vi "onenote_dialog_Fit_image_max_size.vi"(8 "error in (no error)":errorcluster, 10 "image size (pixels)":cluster{"x":i16, "y":i16}, 11 "Picture Refnum":refnum<vi>) -> (0 "error out":errorcluster)   [LabVIEW 2016]
uses:
  <vilib>/Utility/miscctls.llb/LVBoundsTypeDef.ctl
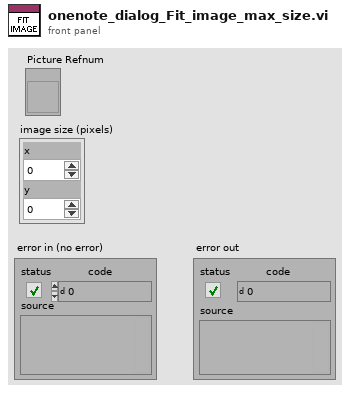
[diagram p1: front panel]
types:
  T1 = typedef "LVBoundsTypeDef.ctl" = cluster{"Width":u32, "Height":u32}
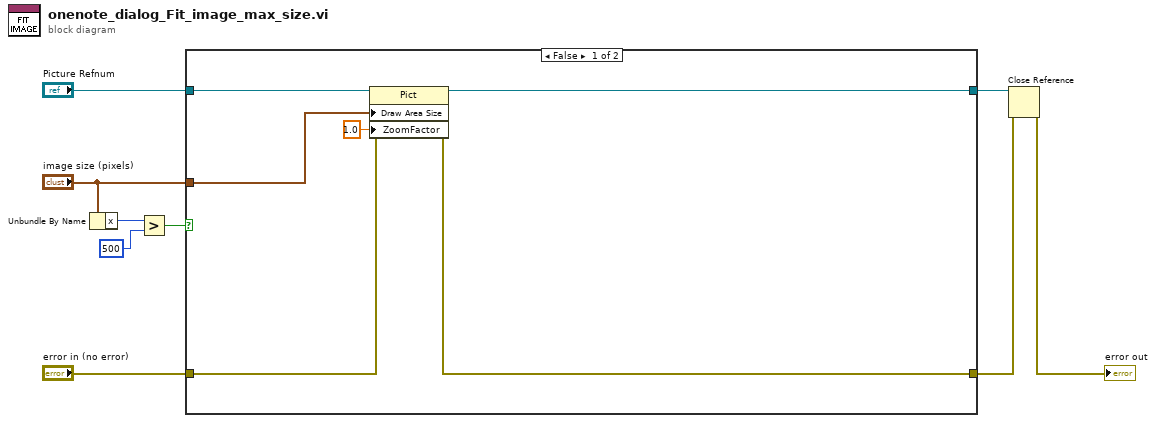
[diagram p0: block diagram]
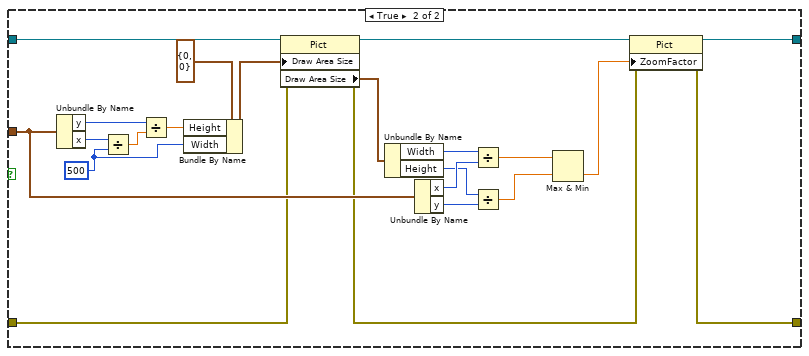
[diagram p2: hidden frame]
diagram:
  n1 = Unbundle By Name("image size (pixels)") -> ("x"=w9:i16)
  n2 = Greater?(x=w9, y=i16 500) -> (0:w7:bool)
  n3 = case shown="False" w7 {
    tunnel: "error in (no error)" -> [w12 w23]
    tunnel: "Picture Refnum" -> [w15 w37]
    tunnel: [w11 w17] -> w1
    tunnel: "image size (pixels)" -> [w14 w29]
    tunnel: [w10 w16] -> w3
    frame False {
      n4 = property class="Pict"(reference=w15, error in=w12, "Draw Area Size"=w14, "ZoomFactor"=sgl 1.0 ("Zoom Factor")) -> (reference out=w10:refnum<vi>, error out=w11:errorcluster)
    }
    frame True {
      w31 = i16 500 ("y")
      n5 = Unbundle By Name(w29) -> ("y"=w34:i16, "x"=w36:i16)
      n6 = Divide(x=w36, y=w31) -> (x/y=w35:dbl)
      n7 = Divide(x=w34, y=w35) -> (x/y=w32:dbl)
      n8 = Bundle By Name(cluster=T1 {"Width"=0, "Height"=0} ("Draw Area Size"), "Height"=w32, "Width"=w31) -> (w30:T1)
      n9 = property class="Pict"(reference=w37, error in=w23, "Draw Area Size"=w30) -> (reference out=w22:refnum<vi>, error out=w18:errorcluster, "Draw Area Size"=w28:T1)
      n10 = Unbundle By Name(w28) -> ("Width"=w26:u32, "Height"=w25:u32)
      n11 = Unbundle By Name(w29) -> ("x"=w27:i16, "y"=w24:i16)
      n12 = Divide(x=w26, y=w27) -> (x/y=w21:dbl)
      n13 = Divide(x=w25, y=w24) -> (x/y=w20:dbl)
      n14 = Max & Min(x=w21, y=w20) -> (min(x,y)=w19:dbl)  [unwired: 1 out]
      n15 = property class="Pict"(reference=w22, error in=w18, "ZoomFactor"=w19) -> (reference out=w16:refnum<vi>, error out=w17:errorcluster)
    }
  }
  n16 = Close Reference(reference=w3, error in (no error)=w1) -> (error out=→"error out":errorcluster)
